vi "Parse Input Command.vi"(8 "Error In":errorcluster, 11 "Command In":string="Set Output Power 100") -> (0 "Error Out":errorcluster, 1 "Value (Dec)":string, 3 "Command Only":string)   [LabVIEW 2018, in "Hitronics.lvlib" / "Hitronics.lvclass"]
uses:
  Hitronics.lvclass
  <vilib>/regexp/Match Regular Expression.xnode
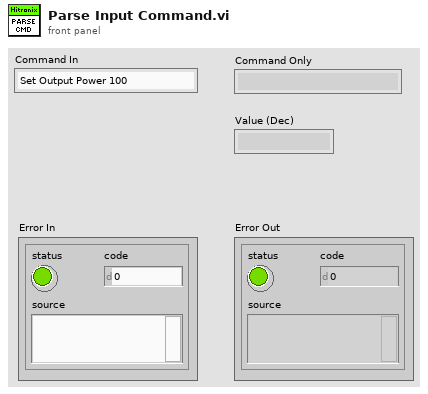
[diagram p1: front panel]
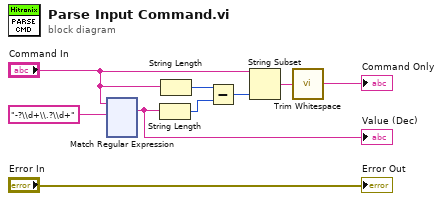
[diagram p0: block diagram]
diagram:
  n1 = xnode "Match Regular Expression"("input string"="Command In", "regular expression"="-?\\d+\\.?\\d+" ("search string")) -> ("whole match"=w5:string)  [unwired: 4 in, 4 out]
  "Value (Dec)" <- w5
  n2 = String Length(string=w5) -> (length=w7:i32)
  n3 = String Length(string="Command In") -> (length=w6:i32)
  n4 = Subtract(x=w6, y=w7) -> (x-y=w8:i32)
  n5 = String Subset(string="Command In", length (rest)=w8) -> (substring=w9:string)  [unwired: 1 in]
  n6 = call <vilib>:"Trim Whitespace.vi"("string"=w9) -> ("trimmed string"=→"Command Only":string)  [unwired: 1 in]
  "Error Out" <- "Error In"
